vi "Chebyshev Window (CDB).vi"(10 "lobe ratio (dB)":dbl=60.0, 11 "X":cdb[](array[numeric])) -> (0 "error":i32, 3 "Windowed X":cdb[](array[numeric]))   [LabVIEW 2020, in "NI_AALPro.lvlib"]
doc: "Applies an asymmetrical Dolph-Chebyshev window to the input sequence <B>X</B>. Wire data to the <B>X</B> input to determine the polymorphic instance to use or manually select the instance."
uses:
  NI_AALPro.lvlib
  <resource>/lvanlys.dll
panel:
  # "Dolph-Chebyshev Window"
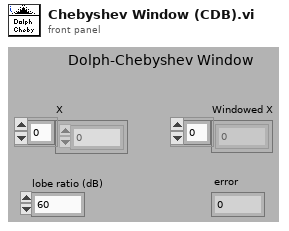
[diagram p1: front panel]
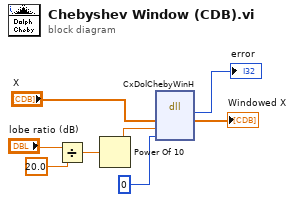
[diagram p0: block diagram]
diagram:
  n1 = Divide(x="lobe ratio (dB)", y=20.0) -> (x/y=w2:dbl)
  n2 = Power Of 10(x=w2) -> (10^x=w3:dbl)
  n3 = dll-call lib="C:/Program Files (x86)/National Instruments/LabVIEW 2020/resource/lvanlys.*" fn="CxDolChebyWinH"("X"="X", "s"=w3, "sym"=0) -> (→"error":i32, "X"=→"Windowed X":cdb[])  [unwired: 5 in, 2 out]
